vi "resistancePIP.vi"(8 "error in (no error)":errorcluster, 11 "Boolean":bool) -> (0 "error out":errorcluster, 3 "RESISTANCE-15":string)   [LabVIEW 2018]
uses:
  Global_usbComm.vi
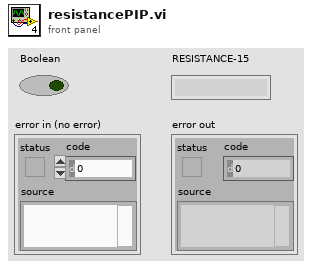
[diagram p1: front panel]
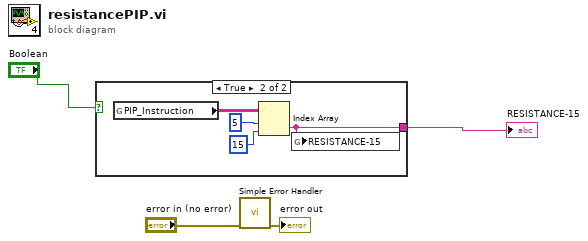
[diagram p0: block diagram]
diagram:
  n1 = case shown="True" "Boolean" {
    tunnel: [_ w5] -> w4
    frame False {
    }
    frame True {
      n2 = global read "Global_usbComm.vi" "PIP_Instruction"() -> (w8:string[][])
      n3 = Index Array(array=w8, index (row)=5, index (col)=15 ("disabled index (col)")) -> (element=w5:string)
      n4 = global write "Global_usbComm.vi" "RESISTANCE-15"(w5) -> ()
    }
  }
  "RESISTANCE-15" <- w4
  n5 = call <vilib>:"Simple Error Handler.vi"("error in (no error)"="error in (no error)") -> ("error out"=→"error out":errorcluster)  [unwired: 4 in, 4 out]
